vi "Read myClass3Array.vi"(8 "error in (no error)":errorcluster, 11 "Class1 in":refnum<class "Class1.lvclass">) -> (0 "error out":errorcluster, 2 "class3Array":refnum<class "Class3.lvclass">[](array[class]), 3 "Class1 out":refnum<class "Class1.lvclass">)   [LabVIEW 2020, in "Class1.lvclass"]
doc: "GCraftsman JSON Object Serialization Toolkit\nwww.GCraftsman.com\nCopyright (c) 2017, GCraftsman"
uses:
  Class1.lvclass
  Class1.lvclass/Class1.ctl
  Class3/Class3.lvclass
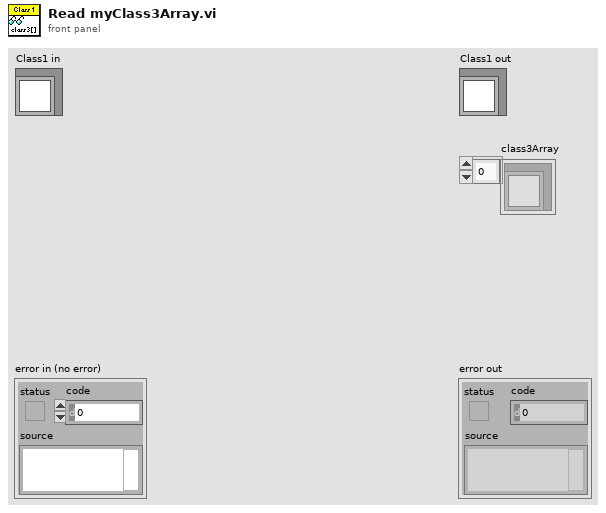
[diagram p1: front panel]
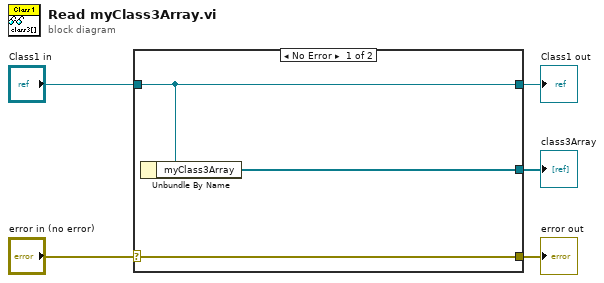
[diagram p0: block diagram]
diagram:
  n1 = case shown="No Error" "error in (no error)" {
    selector: "error in (no error)" -> [w8 w9]
    tunnel: [w8 w9] -> w4
    tunnel: [w7 w10] -> w2
    tunnel: "Class1 in" -> [w7 w10]
    tunnel: [w6 _] -> w1
    frame No Error {
      n2 = Unbundle By Name(w7) -> ("myClass3Array"=w6:refnum<class "Class3.lvclass">[])
    }
    frame Error {
    }
  }
  "error out" <- w4
  "Class1 out" <- w2
  "class3Array" <- w1
